vi "Main5.vi"() -> ()   [LabVIEW 2014]
uses:
  MultiChannelScheduling 1/Enum State Typedef.ctl
  <vilib>/Utility/error.llb/DialogType.ctl
  <vilib>/_DAQmxBase/Internals/DAQmxBase Create Channel (AI-Voltage-Basic).vi
  <vilib>/_DAQmxBase/Internals/DAQmxBase Timing (Sample Clock).vi
  <vilib>/Utility/file.llb/Write To Spreadsheet File (string).vi
  <vilib>/_DAQmxBase/Internals/DAQmxBase Read (Analog 2D DBL NChan NSamp).vi
  <vilib>/Utility/file.llb/Write To Spreadsheet File (DBL).vi
panel:
  in  "Low Pass Filter (Hz)":T1(ring)
  in  "Gain":T2(ring)
  in  "High Pass Filter (Hz)":T3(ring)
  in  "Stop Preview":bool
  in  "OK Button":bool
  in  "Physical channel":tag
  out "State":T4
  in  "Clear Display":bool
  in  "Preview Button":bool
  out "size(s)":i32
  in  "pH":dbl
  in  "Conductivity (mS)":dbl
  out "Iterations Recorded":i32
  in  "Recording Time (seconds)":dbl
  in  "Sample Rate":i32=1000
  in  "Stop Button":bool
  out "Waveform Chart":waveform(dbl)(graph)
  in  "Notch Filter":bool
  in  "Amplifier Model":u16(ring) items=["Select a Model", "AM 1700", "BMA 200"]
  in  "AC/DC Switch":bool
  in  "Temperature (deg C)":dbl
  in  "User Comments":string
  out "Start Time hr/min":string
  out "Date mm/dd/yy":string
  in  "Species":string
  in  "Exit Button":bool
  in  "Record Button":bool
  # "MSU EFISH Lab Single Channel Electronic Pulse Recorder"
  # "Blue for On\nOrange for Off"
  # "DC"
  # "AC"
  # "Blue for AC and Orange for DC"
  # "Must enter numbers into here before you start"
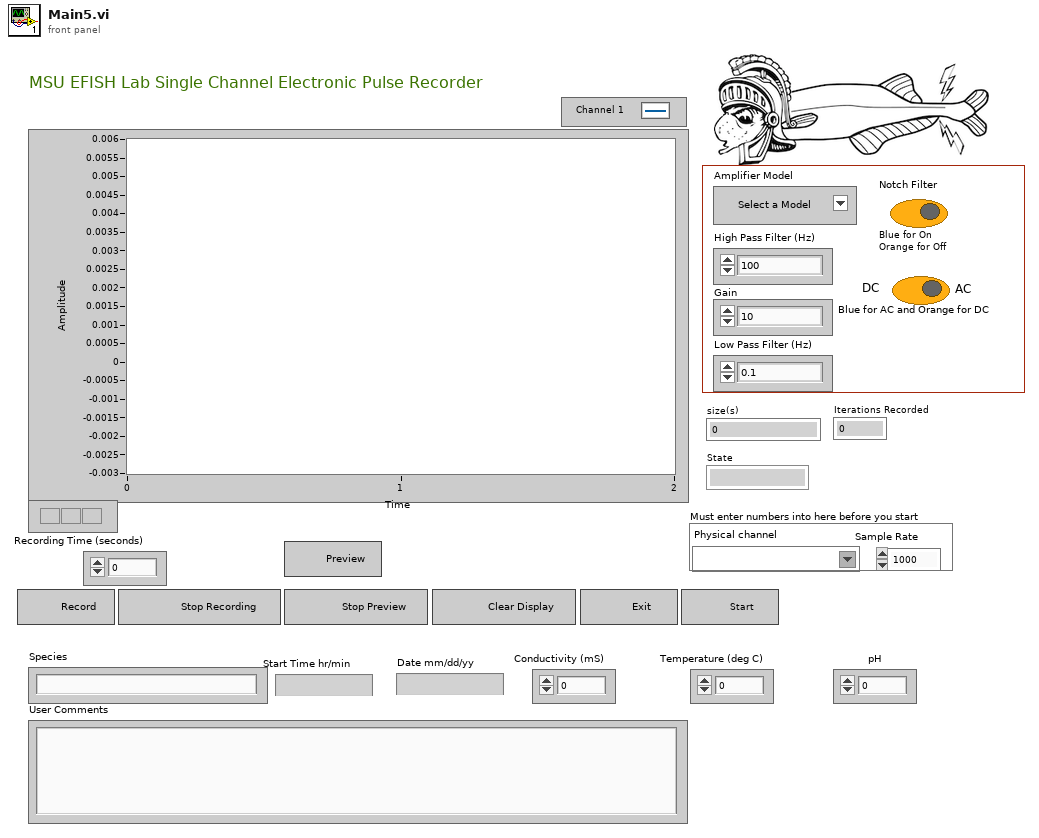
[diagram p1: front panel]
types:
  T1 = enum16{"0.1", "1", "3", "10", "30", "100", "300"}
  T2 = enum16{"10", "20", "50", "100", "200", "500", "1000", "2k", "5k", "10k", "20k", "50k"}
  T3 = enum16{"100", "500", "1000", "3000", "5000", "10,000", "20,000", "30,000", "50,000"}
  T4 = typedef "Enum State Typedef.ctl" = enum16{"", "Open FIle", "Beginning State", "Set the Sample Clock", "Prepreview Handling", "Clear Display", "Preview Data", "Stop", "Exit", "Record", "Create File"}
  T5 = typedef "DialogType.ctl" = u16
  T6 = cluster{"High Pass Filter (Hz)":enum16{"100", "500", "1000", "3000", "5000", "10,000", "20,000", "30,000", "50,000"}, "Gain ":enum16{"10", "20", "50", "100", "200", "500", "1000", "2k", "5k", "10k", "20k", "50k"}, "Low Pass Filter (Hz)":enum16{"0.1", "1", "3", "10", "30", "100", "300"}, "Amplifier Model":u16, "Notch Filter":bool, "AC/DC Switch":bool, "Temperature (deg C)":dbl, "Conductivity (mS)":dbl, "pH":dbl, "User Comments":string, "Species":string}
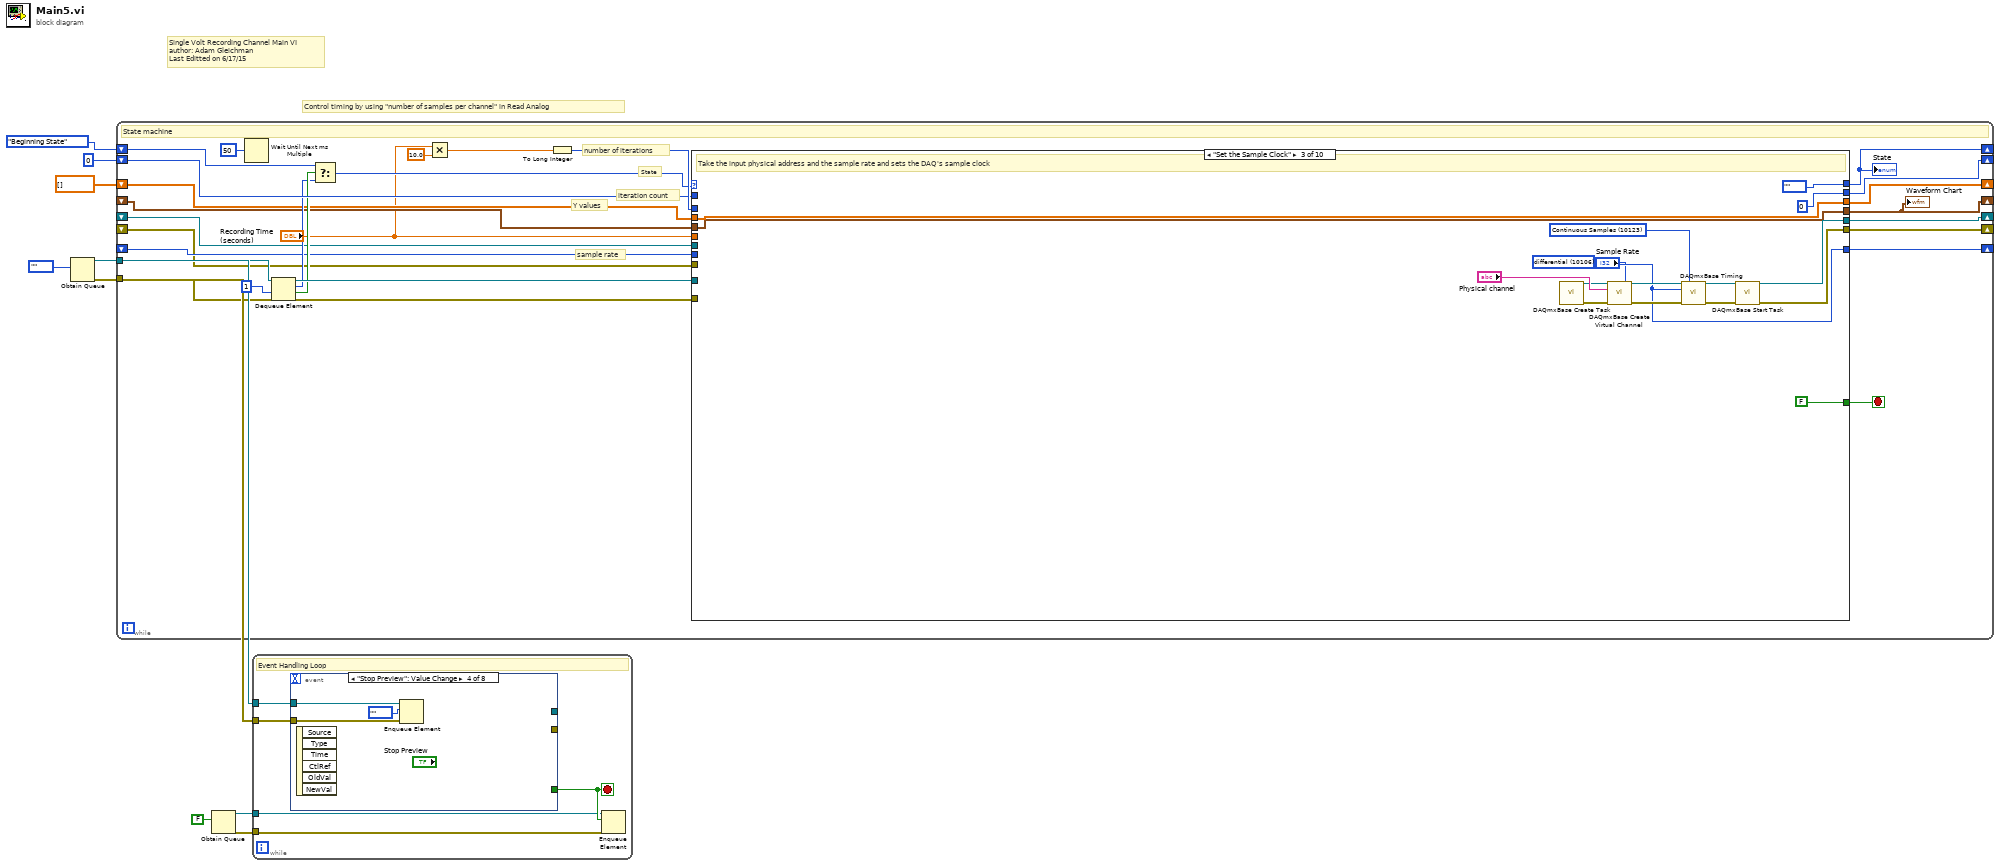
[diagram p0: block diagram]
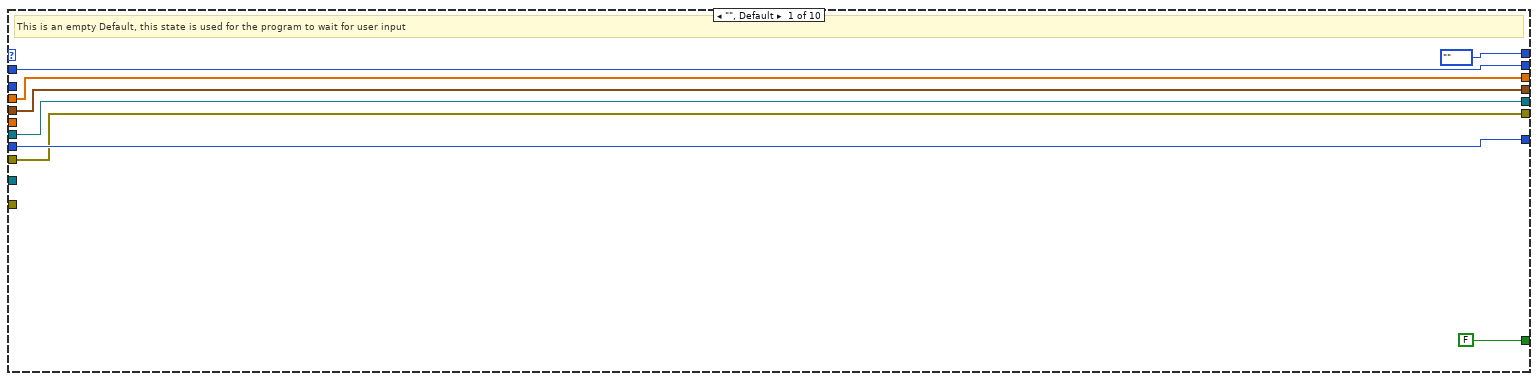
[diagram p2: hidden frame]
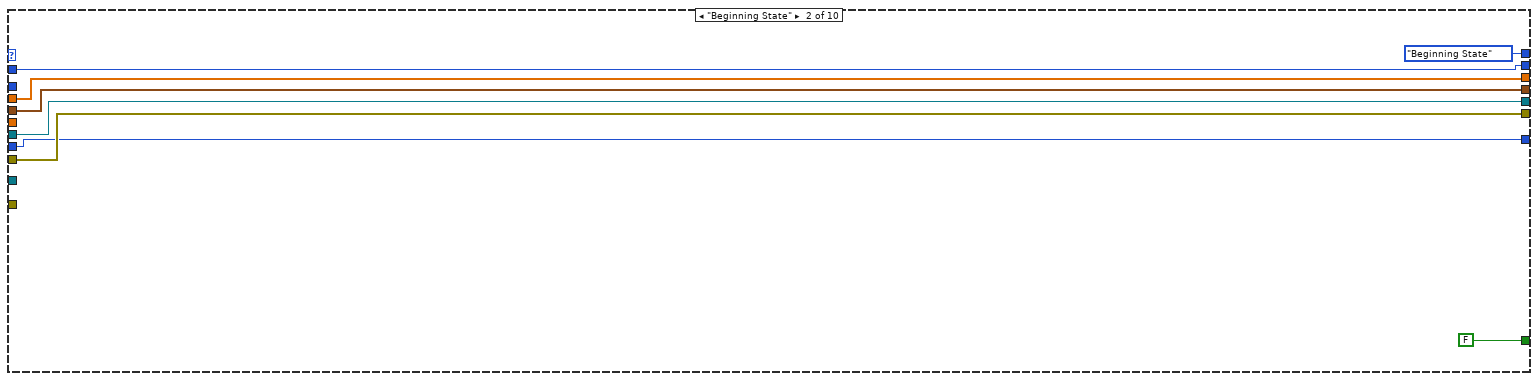
[diagram p3: hidden frame]
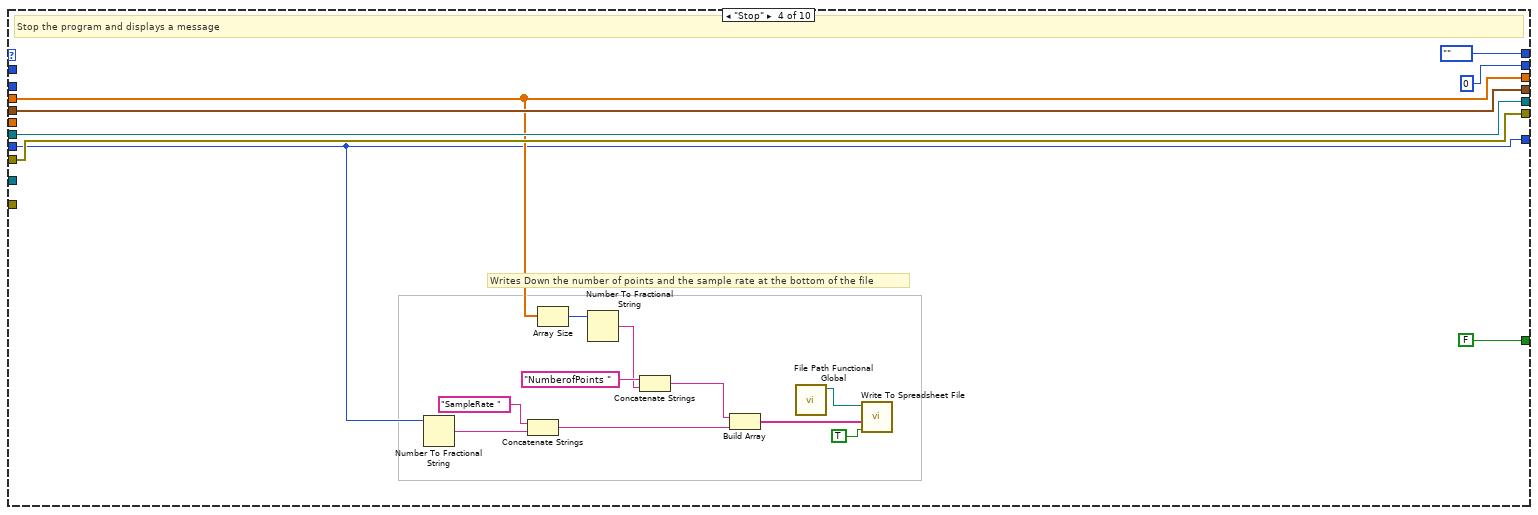
[diagram p4: hidden frame]
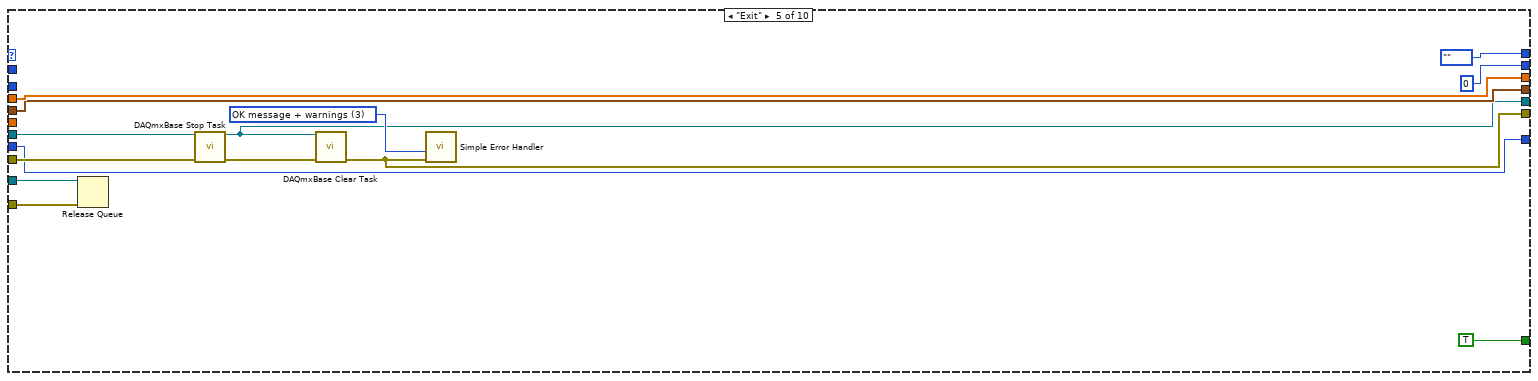
[diagram p5: hidden frame]
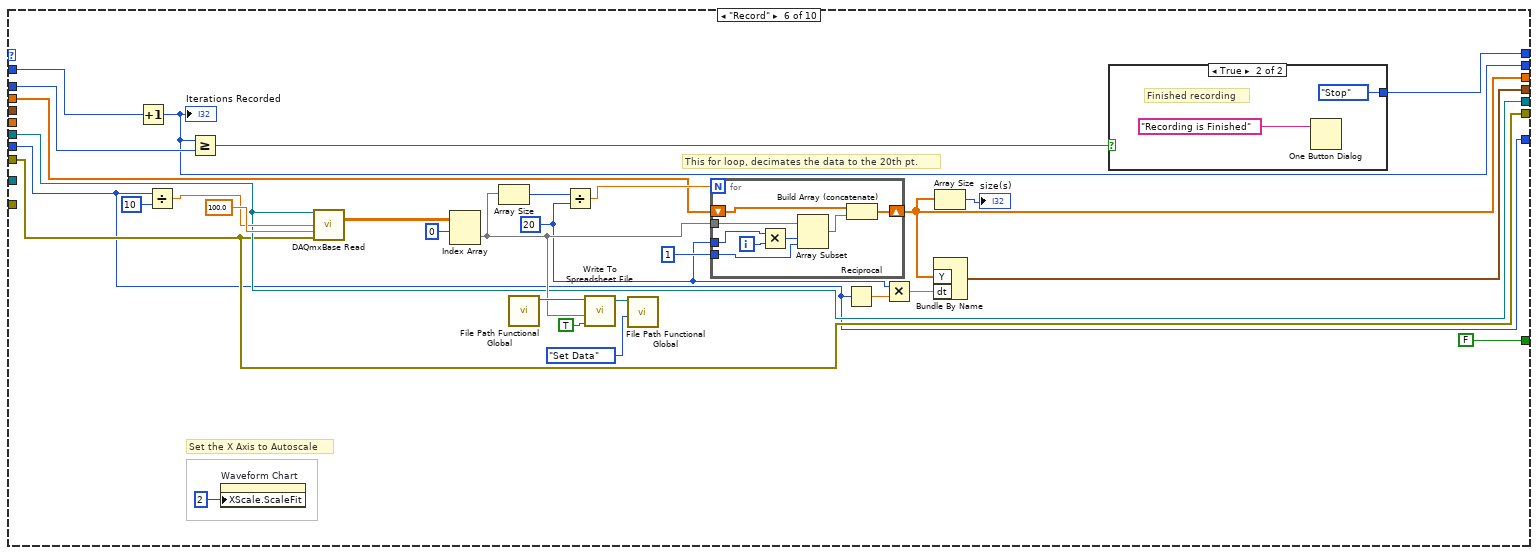
[diagram p6: hidden frame]
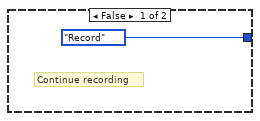
[diagram p7: hidden frame]
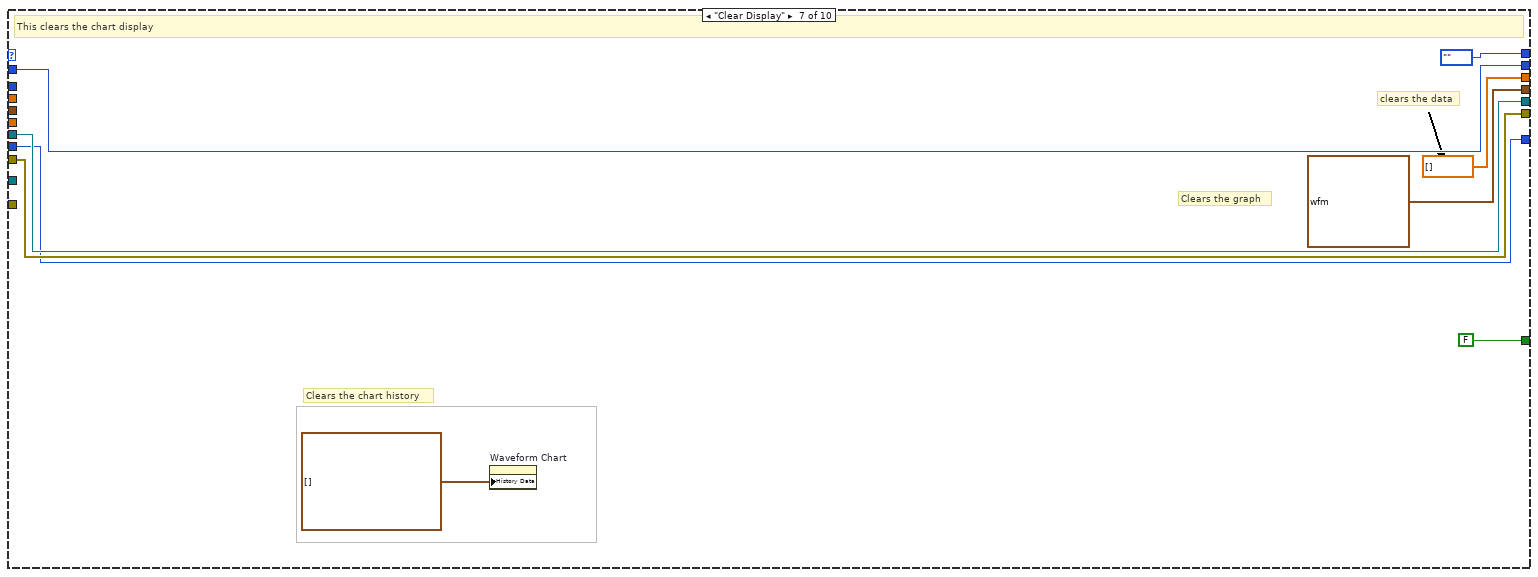
[diagram p8: hidden frame]
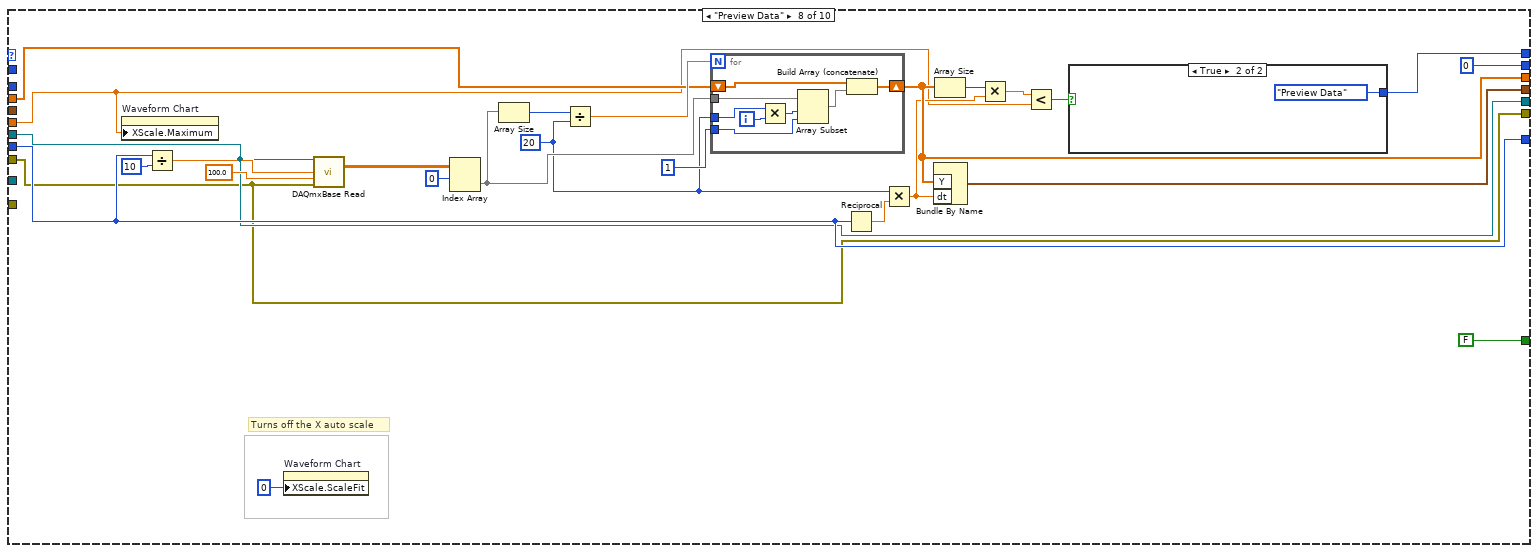
[diagram p9: hidden frame]
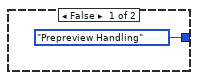
[diagram p10: hidden frame]
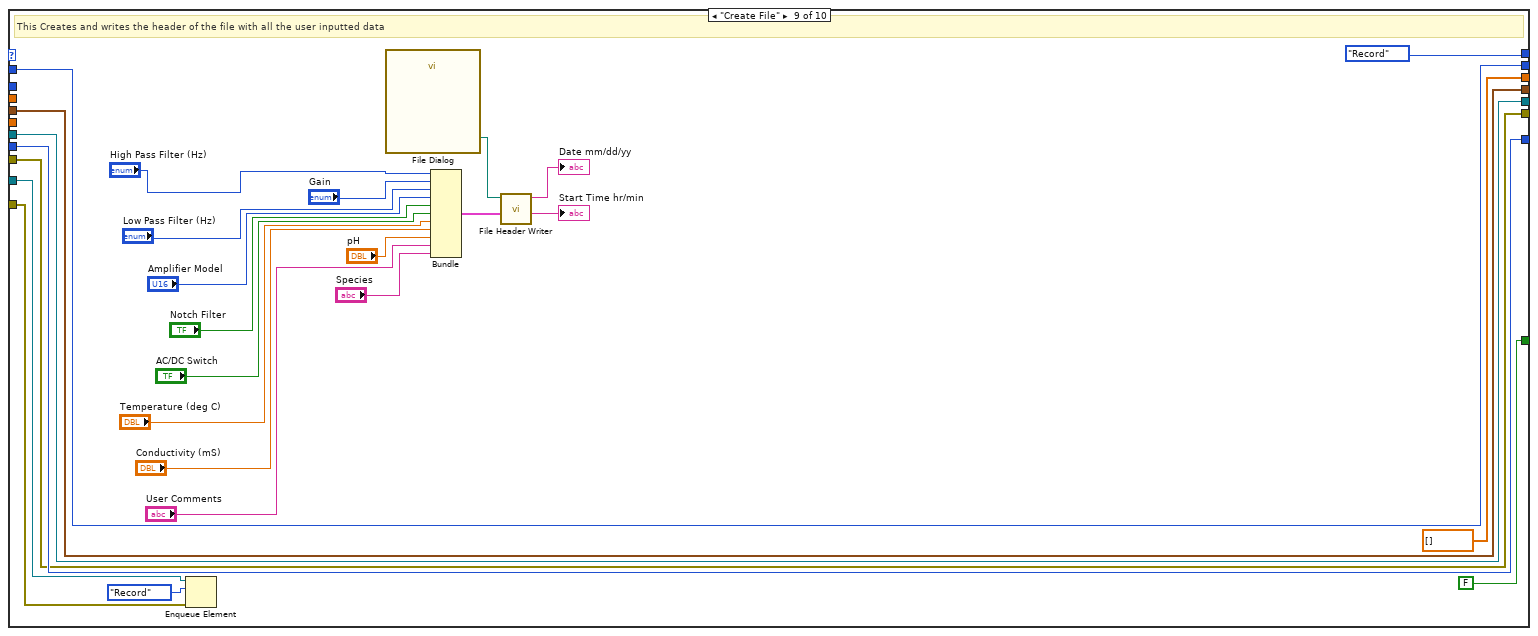
[diagram p11: hidden frame]
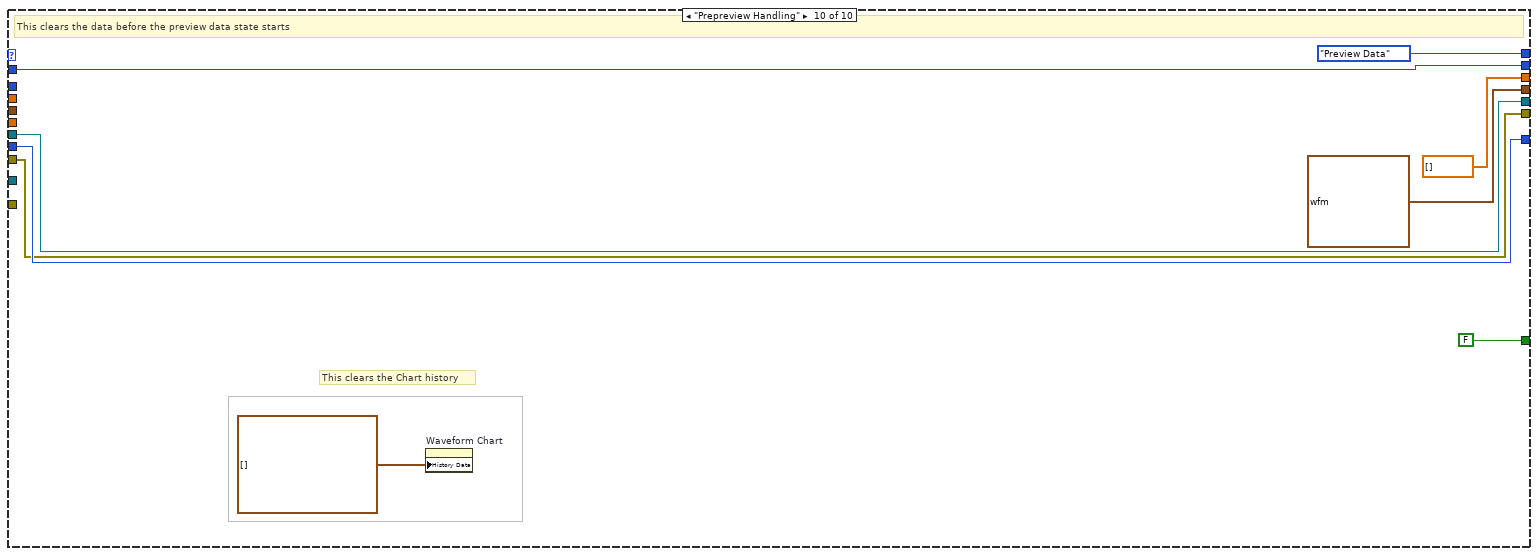
[diagram p12: hidden frame]
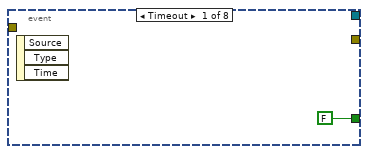
[diagram p13: hidden frame]
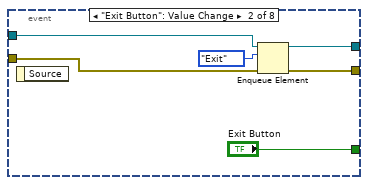
[diagram p14: hidden frame]
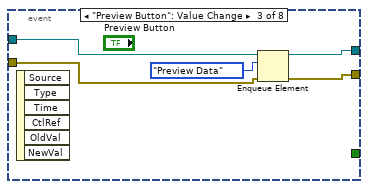
[diagram p15: hidden frame]
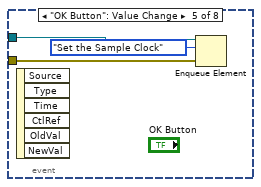
[diagram p16: hidden frame]
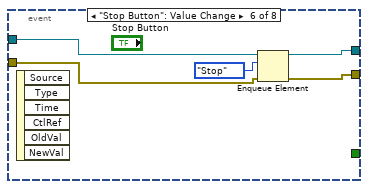
[diagram p17: hidden frame]
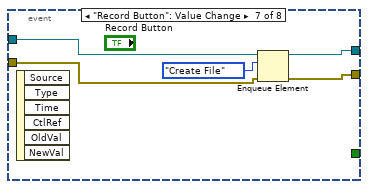
[diagram p18: hidden frame]
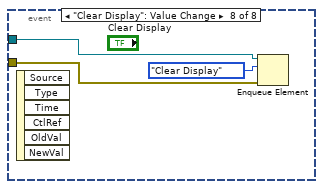
[diagram p19: hidden frame]
diagram:
  # "Single Volt Recording Channel Main VI\nauthor: Adam Gleichman\nLast Editted on 6/17/15"
  # "Control timing by using \"number of samples per channel\" in Read Analog"
  n1 = Obtain Queue(element data type=Enum_State_Typedef."" ("State")) -> (queue out=w8:refnum<queue>, error out=w7:errorcluster)  [unwired: 4 in, 1 out]
  n2 = while {
    tunnel: w8 -> [w37]
    tunnel: w7 -> [w36]
    shift-right: [w29] -> _
    shift-left: 0 -> [w30]
    shift-right: [w24] -> _
    shift-left: Enum_State_Typedef."Beginning State" ("State") -> [w26]
    shift-right: [w22] -> _
    shift-left: _ -> [w23]
    shift-right: [w16] -> _
    shift-left: dbl[] [] -> [w19]
    shift-right: [w18] -> _
    shift-left: _ -> [w17]
    shift-right: [w14] -> _
    shift-left: _ -> [w12]
    shift-right: [w13] -> _
    shift-left: _ -> [w11]
    stop <- w35 stop-if-true
    # "State"
    # "iteration count"
    # "Y values"
    # "sample rate"
    # "number of iterations"
    # "State machine"
    n3 = Wait Until Next ms Multiple(millisecond multiple=u32 50) -> ()  [unwired: 1 out]
    n4 = Dequeue Element(queue=w37, timeout in ms (-1)=1, error in (no error)=w36) -> (queue out=w34:refnum<queue>, element=w27:T4, timed out?=w28:bool, error out=w33:errorcluster)
    n5 = Select(t=w26, s=w28, f=w27) -> (s? t:f=w25:T4)
    n6 = Multiply(x="Recording Time (seconds)", y=10.0) -> (x*y=w10:dbl)
    n7 = To Long Integer(number=w10) -> (32bit integer=w31:i32)
    n8 = case shown="\"Set the Sample Clock\"" w25 {
      tunnel: [FALSE FALSE FALSE FALSE TRUE FALSE FALSE FALSE FALSE FALSE] -> w35
      tunnel: w34 -> [_ _ _ _ w97 _ _ _ w214 _]
      tunnel: w33 -> [_ _ _ _ w96 _ _ _ w213 _]
      tunnel: w12 -> [w39 w49 _ w84 w100 w105 w146 w154 w193 w216]
      tunnel: w11 -> [w38 w50 _ w83 w99 w104 w145 w153 w192 w215]
      tunnel: w23 -> [w42 w47 _ w79 w93 w103 w144 w161 w210 w218]
      tunnel: w31 -> [_ _ _ _ _ w125 _ _ _ _]
      tunnel: w30 -> [w44 w46 _ _ _ w126 w152 _ w211 w219]
      tunnel: [w44 w46 0 ("Sample Rate") 0 0 w120 w152 0 w211 w219] -> w29
      tunnel: [Enum_State_Typedef."" ("State") Enum_State_Typedef."Beginning State" ("State") Enum_State_Typedef."" ("State") Enum_State_Typedef."" ("State") Enum_State_Typedef."" ("State") w122 Enum_State_Typedef."" ("State") w163 Enum_State_Typedef."Record" ("State") Enum_State_Typedef."Preview Data" ("State")] -> w24
      tunnel: [w42 w47 "Sample Rate" w79 w93 w103 w144 w161 w210 w218] -> w22
      tunnel: [w41 w52 w59 w81 w92 w113 dbl[] [] w162 dbl[] [] dbl[] []] -> w16
      tunnel: w19 -> [w41 w52 w59 w81 w92 w112 _ w165 _ _]
      tunnel: [w40 w51 w58 w85 w91 w111 waveform(dbl) {"t0"=timestamp(0 s since 1904-01-01), "dt"=1.0, "Y"=[]} w164 w201 waveform(dbl) {"t0"=timestamp(0 s since 1904-01-01), "dt"=1.0, "Y"=[]}] -> w18
      tunnel: w17 -> [w40 w51 w58 w85 w91 _ _ _ w201 _]
      tunnel: "Recording Time (seconds)" -> [_ _ _ _ _ _ _ w156 _ _]
      tunnel: [w39 w49 w62 w84 w90 w105 w146 w154 w193 w216] -> w14
      tunnel: [w38 w50 w61 w83 w89 w104 w145 w153 w192 w215] -> w13
      frame "", Default {
        # "This is an empty Default, this state is used for the program to wait for user input"
      }
      frame "Beginning State" {
      }
      frame "Set the Sample Clock" {
        w54 = 10106 items=["default"=-1, "differential"=10106, "RSE"=10083, "NRSE"=10078] ("input terminal configuration")
        w65 = 10123 items=["Finite Samples"=10178, "Continuous Samples"=10123, "Hardware Timed Single Point"=12522] ("sample mode")
        # "Take the input physical address and the sample rate and sets the DAQ's sample clock"
        n9 = call <vilib>:"DAQmxBase Create Task.vi"() -> ("task out"=w69:refnum<k21>, "error out"=w68:errorcluster)  [unwired: 14 in]
        n10 = call-poly <vilib>:"DAQmxBase Create Virtual Channel.vi"("task in"=w69, "input terminal configuration"=w54, "physical channels"="Physical channel", "error in"=w68) -> ("task out"=w67:refnum<k21>, "error out"=w66:errorcluster)  [unwired: 10 in]
        n11 = call-poly <vilib>:"DAQmxBase Timing.vi"("task/channels in"=w67, "sample mode"=w65, "rate"="Sample Rate", "error in"=w66) -> ("task out"=w64:refnum<k21>, "error out"=w63:errorcluster)  [unwired: 10 in]
        n12 = call <vilib>:"DAQmxBase Start Task.vi"("task/channels in"=w64, "error in"=w63) -> ("task out"=w62:refnum<k21>, "error out"=w61:errorcluster)  [unwired: 12 in]
      }
      frame "Stop" {
        # "Writes Down the number of points and the sample rate at the bottom of the file"
        # "Stop the program and displays a message"
        n13 = Number To Fractional String(number=w79) -> (F-format string=w78:string)  [unwired: 3 in]
        n14 = Concatenate Strings("SampleRate ", w78) -> (w74:string)
        n15 = Array Size(array=w81) -> (size(s)=w77:i32)
        n16 = Number To Fractional String(number=w77) -> (F-format string=w76:string)  [unwired: 3 in]
        n17 = Concatenate Strings("NumberofPoints " ("string"), w76) -> (w75:string)
        n18 = Build Array(w75, w74) -> (w72:string[])
        n19 = call "File Path Functional Global.vi"() -> ("File Path Output"=w73:path)  [unwired: 11 in]
        n20 = call-poly <vilib>:"Write To Spreadsheet File.vi"("append to file? (new file:F)"=TRUE, "1D data"=w72, "file path (dialog if empty)"=w73) -> ()  [unwired: 5 in, 1 out]
      }
      frame "Exit" {
        w98 = T5 3 items=["no dialog", "OK message", "continue or stop message", "OK message + warnings", "continue/stop + warnings"] ("type of dialog (OK msg:1)")
        n21 = Release Queue(queue=w97, error in (no error)=w96) -> ()  [unwired: 1 in, 3 out]
        n22 = call <vilib>:"DAQmxBase Stop Task.vi"("task/channels in"=w100, "error in"=w99) -> ("task out"=w90:refnum<k21>, "error out"=w101:errorcluster)  [unwired: 12 in]
        n23 = call <vilib>:"DAQmxBase Clear Task.vi"("task in"=w90, "error in"=w101) -> ("error out"=w89:errorcluster)  [unwired: 13 in]
        n24 = call <vilib>:"Simple Error Handler.vi"("type of dialog (OK msg:1)"=w98, "error in (no error)"=w89) -> ()  [unwired: 3 in, 5 out]
      }
      frame "Record" {
        w108 = 20 ("y")
        # "This for loop, decimates the data to the 20th pt."
        # "Set the X Axis to Autoscale"
        n25 = Increment(x=w126) -> (x+1=w120:i32)
        "Iterations Recorded" <- w120
        n26 = Divide(x=w103, y=10) -> (x/y=w123:dbl)
        n27 = Greater Or Equal?(x=w120, y=w125) -> (x >= y?=w121:bool)
        n28 = property on="Waveform Chart" class="WFChart (strict)"("XScale.ScaleFit"=u8 2 ("X Scale.Scale Fit")) -> ()  [unwired: 2 in, 2 out]
        n29 = call-poly <vilib>:"DAQmxBase Read.vi"("task/channels in"=w105, "number of samples per channel"=w123, "timeout"=100.0, "error in"=w104) -> ("data"=w118:dbl[][])  [unwired: 9 in, 2 out]
        n30 = Index Array(array=w118, index (row)=0) -> (element=w110:dbl[])  [unwired: 1 in]
        n31 = Array Size(array=w110) -> (size(s)=w117:i32)
        n32 = call "File Path Functional Global.vi"() -> ("File Path Output"=w130:path)  [unwired: 11 in]
        n33 = Divide(x=w117, y=w108) -> (x/y=w116:dbl)
        n34 = call-poly <vilib>:"Write To Spreadsheet File.vi"("append to file? (new file:F)"=TRUE, "1D data"=w110, "file path (dialog if empty)"=w130) -> ("new file path (Not A Path if cancelled)"=w128:path)  [unwired: 5 in]
        n35 = call "File Path Functional Global.vi"("Enum"=enum16{"Get Data", "Set Data"}."Set Data", "File Path Control"=w128) -> ()  [unwired: 9 in, 1 out]
        n36 = for {
          N: w116 -> [_]
          shift-right: [w133] -> w113
          shift-left: w112 -> [w135]
          tunnel: w110 -> [w140]
          tunnel: w108 -> [w138]
          tunnel: 1 ("y") -> [w136]
          i -> [w139]
          n37 = Multiply(x=w138, y=w139) -> (x*y=w137:i32)
          n38 = Array Subset(array=w140, index=w137, length=w136) -> (w134:dbl[])
          n39 = Build Array (concatenate)(w135, w134) -> (w133:dbl[])
        }
        n40 = Reciprocal(x=w103) -> (1/x=w109:dbl)
        n41 = Multiply(x=w108, y=w109) -> (x*y=w107:dbl)
        n42 = Bundle By Name("Y"=w113, "dt"=w107) -> (w111:waveform(dbl))  [unwired: 1 in]
        n43 = Array Size(array=w113) -> (size(s)=→"size(s)":i32)
        n44 = case shown="True" w121 {
          tunnel: [Enum_State_Typedef."Record" ("State") Enum_State_Typedef."Stop" ("State")] -> w122
          frame False {
            # "Continue recording"
          }
          frame True {
            # "Finished recording"
            n45 = One Button Dialog(message="Recording is Finished") -> ()  [unwired: 1 in, 1 out]
          }
        }
      }
      frame "Clear Display" {
        # "clears the data"
        # "Clears the graph"
        # "Clears the chart history"
        # "This clears the chart display"
        n46 = property on="Waveform Chart" class="WFChart (strict)"("History Data"=waveform(dbl)[] []) -> ()  [unwired: 2 in, 2 out]
      }
      frame "Preview Data" {
        w166 = 20 ("y")
        # "Turns off the X auto scale"
        n47 = property on="Waveform Chart" class="WFChart (strict)"("XScale.Maximum"=w156) -> ()  [unwired: 2 in, 2 out]
        n48 = Divide(x=w161, y=10) -> (x/y=w173:dbl)
        n49 = property on="Waveform Chart" class="WFChart (strict)"("XScale.ScaleFit"=u8 0 ("X Scale.Scale Fit")) -> ()  [unwired: 2 in, 2 out]
        n50 = call-poly <vilib>:"DAQmxBase Read.vi"("task/channels in"=w154, "number of samples per channel"=w173, "timeout"=100.0, "error in"=w153) -> ("data"=w172:dbl[][])  [unwired: 9 in, 2 out]
        n51 = Index Array(array=w172, index (row)=0) -> (element=w168:dbl[])  [unwired: 1 in]
        n52 = Array Size(array=w168) -> (size(s)=w171:i32)
        n53 = Divide(x=w171, y=w166) -> (x/y=w170:dbl)
        n54 = for {
          N: w170 -> [_]
          shift-right: [w181] -> w162
          shift-left: w165 -> [w183]
          tunnel: w168 -> [w188]
          tunnel: w166 -> [w186]
          tunnel: 1 ("y") -> [w184]
          i -> [w187]
          n55 = Multiply(x=w186, y=w187) -> (x*y=w185:i32)
          n56 = Array Subset(array=w188, index=w185, length=w184) -> (w182:dbl[])
          n57 = Build Array (concatenate)(w183, w182) -> (w181:dbl[])
        }
        n58 = Reciprocal(x=w161) -> (1/x=w167:dbl)
        n59 = Multiply(x=w166, y=w167) -> (x*y=w158:dbl)
        n60 = Bundle By Name("Y"=w162, "dt"=w158) -> (w164:waveform(dbl))  [unwired: 1 in]
        n61 = Array Size(array=w162) -> (size(s)=w159:i32)
        n62 = Multiply(x=w159, y=w158) -> (x*y=w157:dbl)
        n63 = Less?(x=w157, y=w156) -> (x < y?=w160:bool)
        n64 = case shown="True" w160 {
          tunnel: [Enum_State_Typedef."Prepreview Handling" ("State") Enum_State_Typedef."Preview Data" ("State")] -> w163
          frame False {
          }
          frame True {
          }
        }
      }
      frame "Create File" {
        # "This Creates and writes the header of the file with all the user inputted data"
        n65 = Enqueue Element(queue=w214, element=Enum_State_Typedef."Record", error in (no error)=w213) -> ()  [unwired: 1 in, 3 out]
        n66 = call "File Dialog"() -> ("selected path"=w198:path)  [unwired: 12 in, 3 out]
        n67 = Bundle("High Pass Filter (Hz)"="High Pass Filter (Hz)", "Gain"="Gain", "Low Pass Filter (Hz)"="Low Pass Filter (Hz)", "Amplifier Model"="Amplifier Model", "Notch Filter"="Notch Filter", "AC/DC Switch"="AC/DC Switch", "Temperature (deg C)"="Temperature (deg C)", "Conductivity (mS)"="Conductivity (mS)", "pH"="pH", "User Comments"="User Comments", "Species"="Species") -> (w197:T6)  [unwired: 1 in]
        n68 = call "File Header Writer.vi"("Data Cluster"=w197, "File Path"=w198) -> ("Start Time hr/min"=→"Start Time hr/min":string, "Date mm/dd/yy"=→"Date mm/dd/yy":string)  [unwired: 8 in]
      }
      frame "Prepreview Handling" {
        # "This clears the Chart history"
        # "This clears the data before the preview data state starts"
        n69 = property on="Waveform Chart" class="WFChart (strict)"("History Data"=waveform(dbl)[] []) -> ()  [unwired: 2 in, 2 out]
      }
    }
    "Waveform Chart" <- w18
    "State" <- w24
  }
  n70 = Obtain Queue(element data type=FALSE) -> (queue out=w2:refnum<queue>, error out=w1:errorcluster)  [unwired: 4 in, 1 out]
  n71 = while {
    tunnel: w8 -> [w228]
    tunnel: w7 -> [w227]
    tunnel: w2 -> [w225]
    tunnel: w1 -> [w224]
    stop <- w226 stop-if-true
    # "Event Handling Loop"
    n72 = event shown="[3] \"Stop Preview\": Value Change" {
      selector: _ -> [_ _ _ _ _ _ _ _]
      dyn-events: _ -> [_ _ _ _ _ _ _ _]
      timeout: _ -> [_ _ _ _ _ _ _ _]
      tunnel: [FALSE ("Exit Button") "Exit Button" _ _ _ _ _ _] -> w226
      tunnel: w228 -> [_ w234 w240 w243 w246 w251 w256 w259]
      tunnel: w227 -> [_ w233 w239 w242 w245 w250 w255 w258]
      tunnel: [_ w232 w237 _ _ w248 w253 _] -> _
      tunnel: [_ w231 w236 _ _ w249 w254 _] -> _
      event Timeout {
        n73 = event-data() -> ()  [unwired: 1 in, 3 out]
      }
      event "Exit Button": Value Change {
        n74 = event-data() -> ()  [unwired: 1 in, 1 out]
        n75 = Enqueue Element(queue=w234, element=Enum_State_Typedef."Exit", error in (no error)=w233) -> (queue out=w232:refnum<queue>, error out=w231:errorcluster)  [unwired: 1 in, 1 out]
      }
      event "Preview Button": Value Change {
        n76 = event-data() -> ()  [unwired: 1 in, 6 out]
        n77 = Enqueue Element(queue=w240, element=Enum_State_Typedef."Preview Data", error in (no error)=w239) -> (queue out=w237:refnum<queue>, error out=w236:errorcluster)  [unwired: 1 in, 1 out]
      }
      event "Stop Preview": Value Change {
        n78 = event-data() -> ()  [unwired: 1 in, 6 out]
        n79 = Enqueue Element(queue=w243, element=Enum_State_Typedef."", error in (no error)=w242) -> ()  [unwired: 1 in, 3 out]
      }
      event "OK Button": Value Change {
        n80 = event-data() -> ()  [unwired: 1 in, 6 out]
        n81 = Enqueue Element(queue=w246, element=Enum_State_Typedef."Set the Sample Clock", error in (no error)=w245) -> ()  [unwired: 1 in, 3 out]
      }
      event "Stop Button": Value Change {
        n82 = event-data() -> ()  [unwired: 1 in, 6 out]
        n83 = Enqueue Element(queue=w251, element=Enum_State_Typedef."Stop", error in (no error)=w250) -> (queue out=w248:refnum<queue>, error out=w249:errorcluster)  [unwired: 1 in, 1 out]
      }
      event "Record Button": Value Change {
        n84 = event-data() -> ()  [unwired: 1 in, 6 out]
        n85 = Enqueue Element(queue=w256, element=Enum_State_Typedef."Create File", error in (no error)=w255) -> (queue out=w253:refnum<queue>, error out=w254:errorcluster)  [unwired: 1 in, 1 out]
      }
      event "Clear Display": Value Change {
        n86 = event-data() -> ()  [unwired: 1 in, 6 out]
        n87 = Enqueue Element(queue=w259, element=Enum_State_Typedef."Clear Display", error in (no error)=w258) -> ()  [unwired: 1 in, 3 out]
      }
    }
    n88 = Enqueue Element(queue=w225, element=w226, error in (no error)=w224) -> ()  [unwired: 1 in, 3 out]
  }
